vi "Event Software.vi"(8 "error in (no error)":errorcluster, 11 "[MV] Key Generator in":refnum<class "[MV] Key Generator.lvclass">) -> (0 "error out":errorcluster, 3 "[MV] Key Generator out":refnum<class "[MV] Key Generator.lvclass">)   [LabVIEW 2020, in "[MV] Key Generator.lvlib" / "[MV] Key Generator.lvclass"]
uses:
  [MV] Key Generator.lvclass
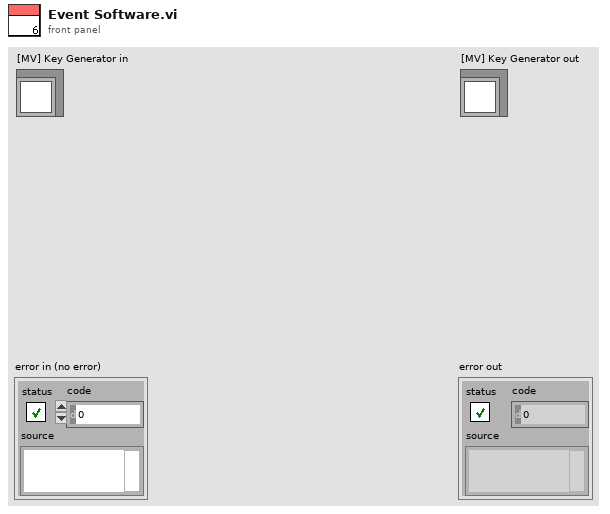
[diagram p1: front panel]
types:
  T1 = map{string, cluster{"private":string, "public":string}}
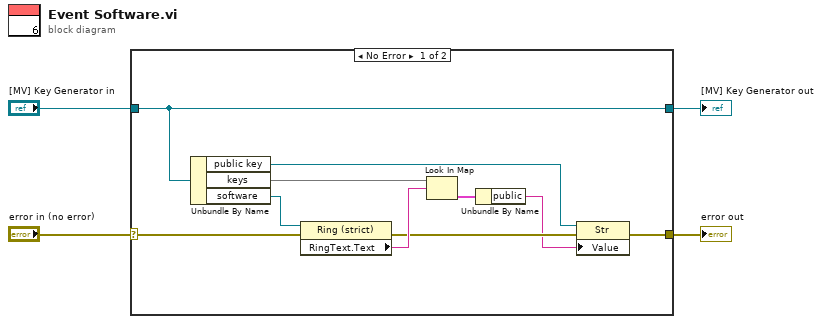
[diagram p0: block diagram]
diagram:
  n1 = case shown="No Error" "error in (no error)" {
    selector: "error in (no error)" -> [w13 w16]
    tunnel: [w5 w16] -> w3
    tunnel: [w14 w15] -> w1
    tunnel: "[MV] Key Generator in" -> [w14 w15]
    frame No Error {
      n2 = Unbundle By Name(w14) -> ("public key"=w7:refnum<vi>, "keys"=w11:T1, "software"=w12:refnum<vi>)
      n3 = property class="Ring (strict)"(reference=w12, error in=w13) -> (error out=w8:errorcluster, "RingText.Text"=w10:string)  [unwired: 1 out]
      n4 = Look In Map(map=w11, key=w10) -> (value=w9:cluster{"private":string, "public":string})  [unwired: 1 in, 1 out]
      n5 = Unbundle By Name(w9) -> ("public"=w6:string)
      n6 = property class="Str"(reference=w7, error in=w8, "Value"=w6) -> (error out=w5:errorcluster)  [unwired: 1 out]
    }
    frame Error {
    }
  }
  "error out" <- w3
  "[MV] Key Generator out" <- w1
